vi "SV TDMS Read Even-Angle Signal (1 Ch).vi"(0 "tdms file":refnum<k34>, 5 "group name in":string="Even-Angle_Signal", 7 "channel name in":string="Channel0", 11 "error in":errorcluster) -> (4 "tdms file out":refnum<k34>, 6 "group name out":string, 8 "channel name out":string, 10 "even-angle signal":cluster{"r0":dbl, "dr":dbl, "Y":dbl[]}={"r0"=0.0, "dr"=1.0, "Y"=[]} {"r0" format="%.2p"; "dr" format="%.2p"; "Y" format="%.2f"}, 12 "even-angle position info":T1, 13 "even-angle channel info":T2={"channel name"="", "description"="", " channel info"={"sensor sensitivity"=1000.0, "engineering units"=1, "dB reference"=1.0, "custom label"="EU", "weighting filter"=0, "pregain"=0.0}} {"channel info"."pregain" format="%.2f"; "channel info"."weighting filter" items=["Linear", "A-weighting", "B-weighting", "C-weighting", "ITU-R 468-4", "Dolby", "CCITT", "C-message", "Wb", "Wc", "Wd", "We", "Wf", "Wh", "Wj", "Wk", "Wm", "AES17 20 kHz lowpass", "AES17 40 kHz lowpass", "AES17 20 kHz highpass", "AES17 40 kHz highpass"]; "channel info"."dB reference" format="%^.1e"; "channel info"."engineering units" items=["custom..."=0, "V"=1, "A"=21, "C"=30, "pC"=31, "s"=32, "-"=29, "Pa"=2, "N"=20, "g"=3, "m/s^2"=4, "m/s"=5, "m"=6, "mm/s"=12, "mm"=13, "micron/s"=14, "micron"=15, "in/s^2"=7, "in/s"=8, "in"=9, "mil/s"=10, "mil"=11, "rad/s^2"=16, "rad/s"=17, "rad"=18, "deg/s^2"=26, "deg/s"=27, "deg"=28, "RPM"=22, "cycle/s^2"=23, "Hz"=24, "cycle"=25, "strain"=19]; "channel info"."sensor sensitivity" format="%#_5f"}, 15 "error out":errorcluster)   [LabVIEW 2017]
doc: "Reads the specified .tdms file and returns data in a format specific to the polymorphic instance selected."
uses:
  <vilib>/addons/_NISVFA/_Shared subVIs/Controls/svc_Resampled Channel Info.ctl
  <vilib>/addons/_NISVFA/_Shared subVIs/Controls/svc_Channel Info.ctl
  <vilib>/addons/_NISVFA/_Shared subVIs/Controls/svc_Engineering Units Text Ring.ctl
  <vilib>/addons/_NISVFA/_Shared subVIs/Controls/svc_Weighting Filter Text Ring.ctl
  <vilib>/addons/_NISVFA/_Shared subVIs/Controls/svc_Position Info.ctl
  <vilib>/addons/_NISVFA/_Shared subVIs/Controls/NI Channel Properties.ctl
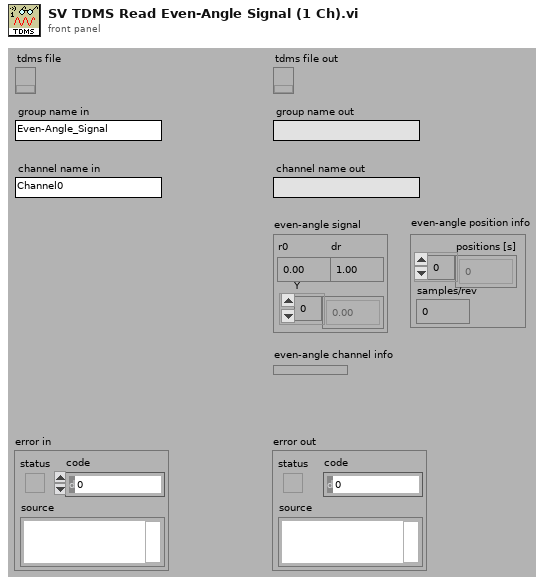
[diagram p1: front panel]
types:
  T1 = typedef "svc_Position Info.ctl" = cluster{"positions [s]":dbl[], "samples/rev":dbl}
  T2 = typedef "svc_Resampled Channel Info.ctl" = cluster{"channel name":string, "description":string, " channel info":T3}
  T3 = typedef "svc_Channel Info.ctl" = cluster{"sensor sensitivity":dbl, "engineering units":T4, "dB reference":dbl, "custom label":string, "weighting filter":T5, "pregain":dbl}
  T4 = typedef "svc_Engineering Units Text Ring.ctl" = u16
  T5 = typedef "svc_Weighting Filter Text Ring.ctl" = u16
  T6 = typedef "NI Channel Properties.ctl" = u16
  T7 = cluster{"property values":dbl, "property values":dbl, "Y":dbl[]}
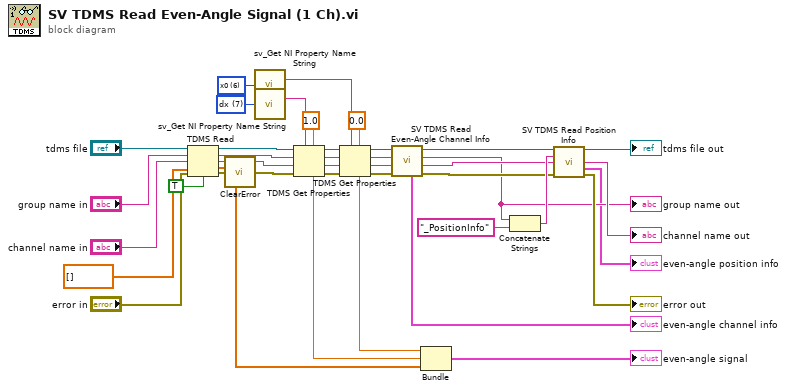
[diagram p0: block diagram]
diagram:
  w30 = T6 6 items=["Channel name", "Channel description", "Y-axis label", "Y-axis unit string", "X-axis label", "X-axis unit string", "x0", "dx", "Number of samples", "X channel", "Filter settled", "dB reference", "Window", "Window parameter", "Window size", "FFT size", "Peak units", "Spectrum type", "Magnitude scale", "Spectral density", "Sensor sensitivity (mV/EU)", "X-axis domain", "LabVIEW datatype"] ("property")
  w31 = T6 7 items=["Channel name", "Channel description", "Y-axis label", "Y-axis unit string", "X-axis label", "X-axis unit string", "x0", "dx", "Number of samples", "X channel", "Filter settled", "dB reference", "Window", "Window parameter", "Window size", "FFT size", "Peak units", "Spectrum type", "Magnitude scale", "Spectral density", "Sensor sensitivity (mV/EU)", "X-axis domain", "LabVIEW datatype"] ("property")
  n1 = TDMS Read(0:"tdms file", 5:"group name in", 7:"channel name in", 11:"error in", 12:dbl[] [] ("Y"), 13:TRUE ("return channels in file order? (F)")) -> (4:w19:refnum<k34>, 6:w17:string, 8:w18:string, 10:w15:dbl[], 15:w2:errorcluster)  [unwired: 2 in, 1 out]
  n2 = call <vilib>:"ClearError.vi"("error in (no error)"=w2) -> ("error out"=w16:errorcluster)
  n3 = call <vilib>:"sv_Get NI Property Name String.vi"("property"=w30) -> ("TDMS property name"=w28:string)  [unwired: 13 in, 1 out]
  n4 = call <vilib>:"sv_Get NI Property Name String.vi"("property"=w31) -> ("TDMS property name"=w29:string)  [unwired: 13 in, 1 out]
  n5 = TDMS Get Properties(5:1.0 ("property values"), 7:w29, 8:w16, 9:w18, 10:w17, 11:w19) -> (0:w32:errorcluster, 1:w33:string, 2:w34:string, 3:w35:refnum<k34>, 4:w22:dbl)  [unwired: 1 out]
  n6 = TDMS Get Properties(5:0.0 ("property values"), 7:w28, 8:w32, 9:w33, 10:w34, 11:w35) -> (0:w37:errorcluster, 1:w39:string, 2:w38:string, 3:w36:refnum<k34>, 4:w23:dbl)  [unwired: 1 out]
  n7 = call <vilib>:"SV TDMS Read Even-Angle Channel Info.vi"("error in"=w37, "channel name in"=w39, "group name in"=w38, "tdms file"=w36) -> ("error out"=w7:errorcluster, "channel name out"=w10:string, "group name out"=w4:string, "tdms file out"=w11:refnum<k34>, "even-angle channel info"=→"even-angle channel info":T2)  [unwired: 2 in, 1 out]
  "group name out" <- w4
  n8 = Bundle("property values"=w23, "property values"=w22, "Y"=w15) -> (→"even-angle signal":T7)  [unwired: 1 in]
  n9 = Concatenate Strings(w4, "_PositionInfo") -> (w12:string)
  n10 = call <vilib>:"SV TDMS Read Position Info.vi"("tdms file"=w11, "group name in"=w12, "channel name in"=w10, "error in"=w7) -> ("tdms file out"=→"tdms file out":refnum<k34>, "channel name out"=→"channel name out":string, "position info"=→"even-angle position info":T1, "error out"=→"error out":errorcluster)  [unwired: 7 in, 1 out]
